vi "Self Starting Simple Frequency Reader.vi"(8 "error in (no error)":errorcluster) -> (0 "error out":errorcluster)   [LabVIEW 2018, in "S3DK.lvlib"]
uses:
  <vilib>/S3DK.lvlib
  <vilib>/Platform/TimedLoop/XDataNode/timing_clust.ctl
  <vilib>/Platform/TimedLoop/XDataNode/nitl_modes.ctl
  <vilib>/Platform/TimedLoop/XDataNode/wakeup.ctl
  <vilib>/platform/TimedLoop/XDataNode/XDataNode.xnode
  <vilib>/Platform/TimedLoop/XDataNode/XDNodeRunTimeDep.lvlib
  .S3DK - Copy/PMU Recorder Light/PMU Recorder Light.lvlib
panel:
  out "Waveform Chart":waveform(sgl)[](graph)
  in  "Quit":bool
  in  "Refresh Rate":i64(ring)=200 items=["50 Hz"=20, "20 Hz"=50, "10 Hz"=100, "5 Hz"=200, "2 Hz"=500, "1 Hz"=1000, "Every 2 sec"=2000, "Every 5 sec"=5000, "Every 10 sec"=10000, "Every minute"=60000]
  # "INPUT"
  # "INTERMEDIATE"
  # "OUTPUT"
  # "USAGE:  Press play. The VI will start the PRL itself and wait for the connection to be established.\n(you will still need to configure the PRL first. If the Simple Frequency Reader works, then this works)"
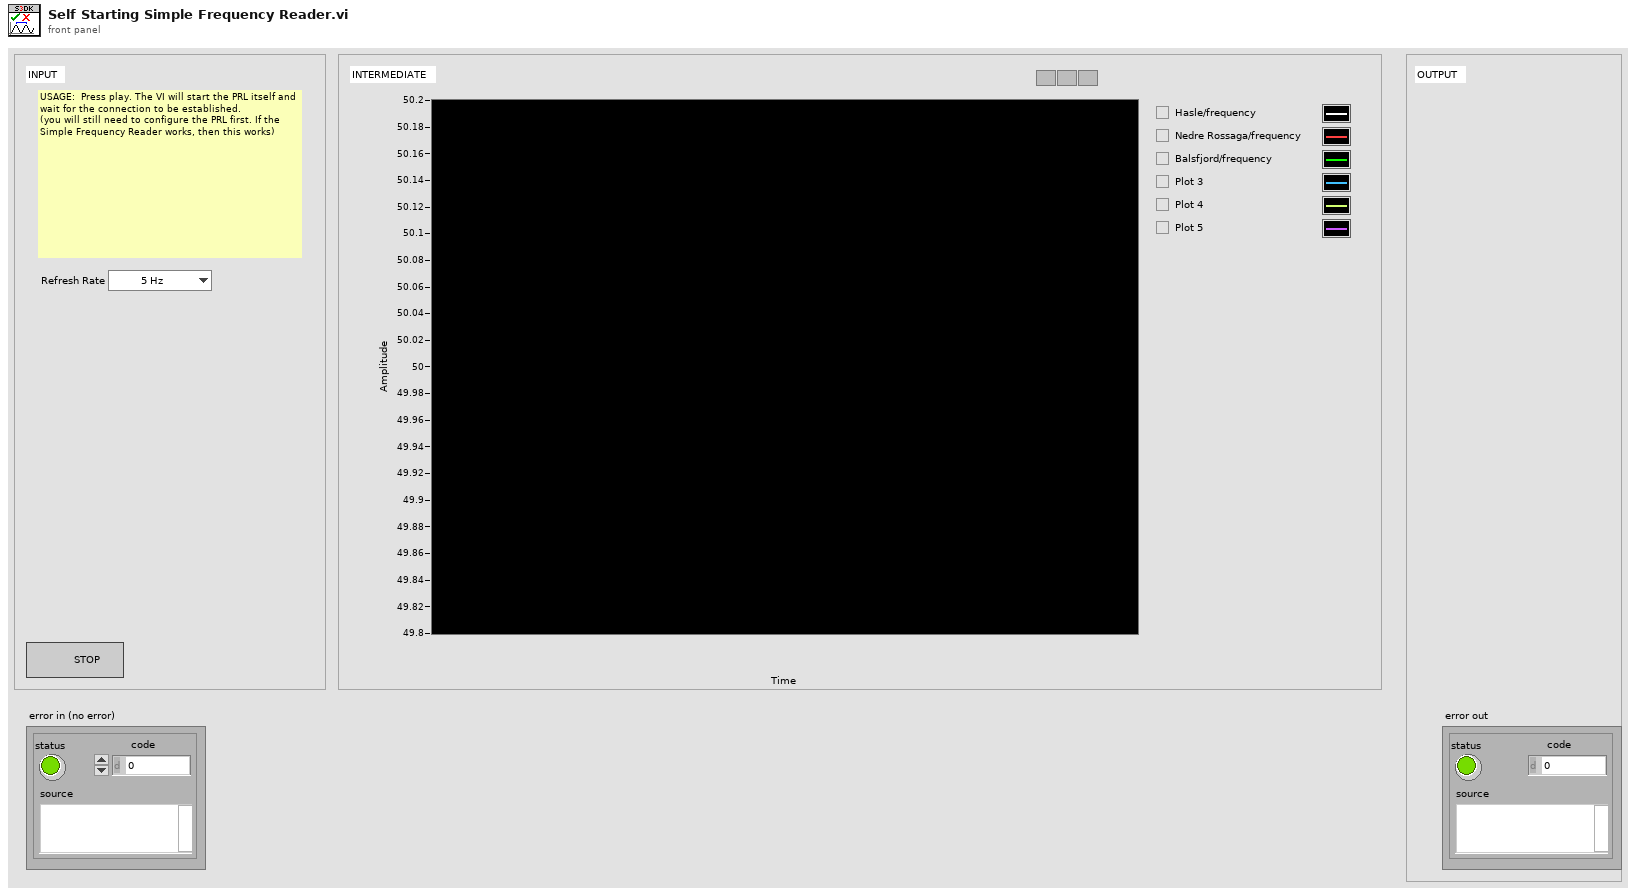
[diagram p1: front panel]
types:
  T1 = enum16{"Run", "Startup", "Get Status", "Pause", "Continue", "Shutdown", "Abort", "Open Panel", "Close Panel"}
  T2 = enum16{"Filter Signals", "Get All Signal Names", "Select Signals on Name", "Select Frequency Only", "Get Selected Signal Names"}
  T3 = typedef "XDNodeRunTimeDep.lvlib/timing_clust.ctl" = cluster{"Expected End [f-1]":u64, "Actual End [f-1]":u64, "Finished Late? [f-1]":bool, "Expected End [i-1]":u64, "Actual End [i-1]":u64, "Finished Late? [i-1]":bool, "Expected Start [i]":u64, "Actual Start [i]":u64, "Expected Start [f]":u64, "Actual Start [f]":u64, "Source Name":string, "Structure Name":string, "Period":i64, "Deadline":i64, "Offset":i64, "Start":i64, "Priority":i32, "Timeout":i32, "Mode":T4, "Wakeup Reason":T5, "Error":errorcluster, "Source Type":string, "Secondary Source Type":string, "Global End Time":u64, "Global Start Time":u64, "Frame Duration":u64, "Iteration Duration":u64, "Assigned CPU":i32, "I/O Scan Engine Mode":u32}
  T4 = typedef "XDNodeRunTimeDep.lvlib/nitl_modes.ctl" = enum32{"No Change", "Process missed periods, maintain original phase", "Discard missed periods, maintain original phase", "Process missed periods, ignore original phase", "Discard missed periods, ignore original phase"}
  T5 = typedef "XDNodeRunTimeDep.lvlib/wakeup.ctl" = enum32{"Normal", "Aborted", "Asynchronous wakeup", "Timing source error", "Timed loop error", "Timeout"}
  T6 = cluster{"Phasor":string[], "Analog":string[], "Digital":string[]}
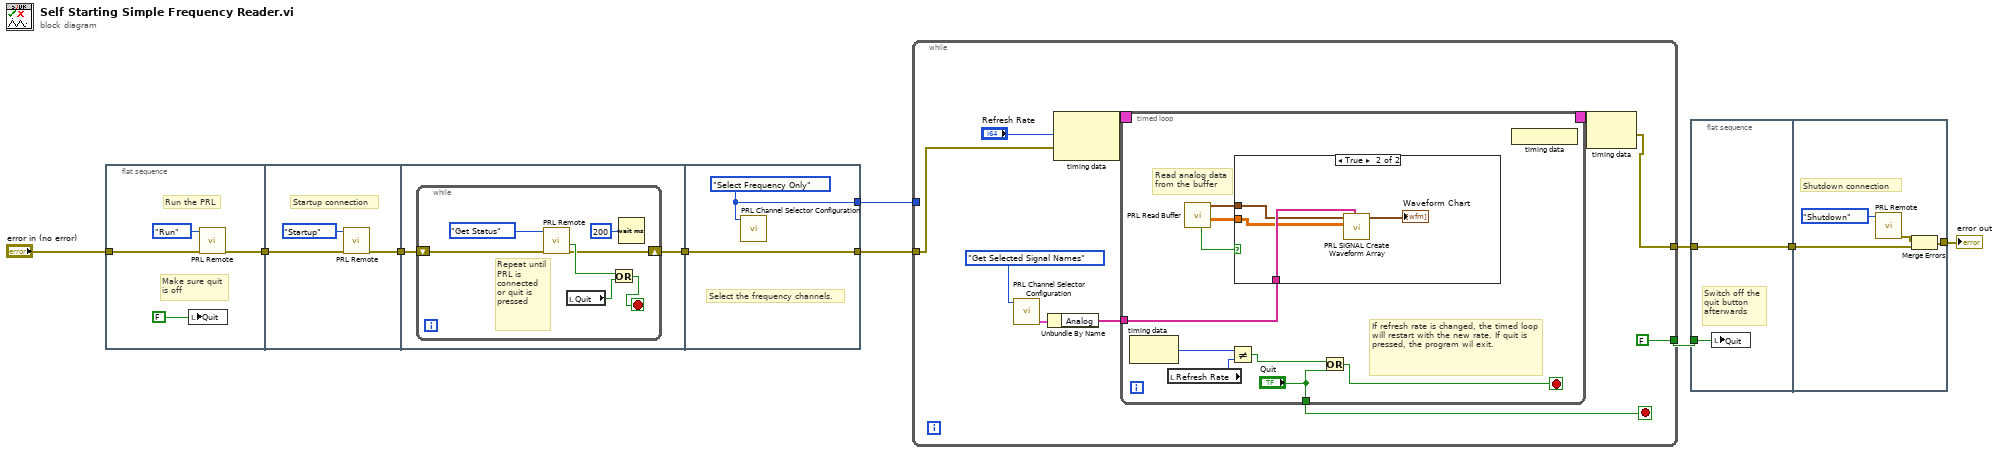
[diagram p0: block diagram]
diagram:
  n1 = flat-sequence {
    tunnel: "error in (no error)" -> [w12]
    tunnel: [w11] -> w7
    tunnel: w7 -> [w16]
    tunnel: [w15] -> w6
    tunnel: w6 -> [w19]
    tunnel: [w18] -> w5
    tunnel: [w28] -> w9
    tunnel: w5 -> [w27]
    tunnel: [w27] -> w4
    frame #0 {
      # "Make sure quit\nis off"
      # "Run the PRL"
      n2 = local write "Quit"(FALSE ("Quit")) -> ()
      n3 = call "PRL Remote.vi"("error in (no error)"=w12, "Action"=T1."Run") -> ("error out"=w11:errorcluster)  [unwired: 4 in, 5 out]
    }
    frame #1 {
      # "Startup connection"
      n4 = call "PRL Remote.vi"("error in (no error)"=w16, "Action"=T1."Startup") -> ("error out"=w15:errorcluster)  [unwired: 4 in, 5 out]
    }
    frame #2 {
      n5 = while {
        shift-right: [w20] -> w18
        shift-left: w19 -> [w21]
        stop <- w24 stop-if-true
        # "Repeat until PRL is connected or quit is pressed"
        n6 = call "PRL Remote.vi"("error in (no error)"=w21, "Action"=T1."Get Status") -> ("error out"=w20:errorcluster, "Connected"=w22:bool)  [unwired: 4 in, 4 out]
        n7 = local read "Quit"() -> (w23:bool)
        n8 = Or(x=w22, y=w23) -> (x .or. y?=w24:bool)
        n9 = Wait (ms)(milliseconds to wait=u32 200) -> ()  [unwired: 1 out]
      }
    }
    frame #3 {
      w28 = T2."Select Frequency Only" ("Action")
      # "Select the frequency channels."
      n10 = call "PRL Channel Selector Configuration.vi"("Action"=w28) -> ()  [unwired: 10 in, 1 out]
    }
  }
  n11 = while {
    tunnel: [FALSE ("Quit")] -> w10
    tunnel: w9 -> [_]
    tunnel: w4 -> [w30]
    tunnel: [w29] -> w2
    stop <- w38 stop-if-true
    n12 = call "PRL Channel Selector Configuration.vi"("Action"=T2."Get Selected Signal Names") -> ("Signal Names Out"=w32:T6)  [unwired: 10 in]
    n13 = Unbundle By Name(w32) -> ("Analog"=w31:string[])
    n14 = node-c288("Refresh Rate", w30) -> (w36:T3)
    n15 = timed-loop {
      timing: w36 -> [_]
      timing-out: [_] -> w35
      tunnel: ["Quit"] -> w38
      tunnel: w31 -> [w39]
      stop <- w45 stop-if-true
      # "Read analog data\nfrom the buffer"
      # "If refresh rate is changed, the timed loop will restart with the new rate. If quit is pressed, the program wil exit."
      n16 = node-c288() -> (w47:i64)  [unwired: 1 in]
      n17 = local read "Refresh Rate"() -> (w46:i64)
      n18 = call "PRL Read Buffer .vi"() -> ("Analog Signals"=w40:sgl[][], "Timestamp"=w41:timestamp[], "Has Data"=w42:bool)  [unwired: 6 in, 3 out]
      n19 = Not Equal?(x=w47, y=w46) -> (x != y?=w44:bool)
      n20 = case shown="True" w42 {
        tunnel: w41 -> [_ w50]
        tunnel: w40 -> [_ w49]
        tunnel: w39 -> [_ w51]
        frame False {
          # "If there is no new data there is no point in sending them to the plot."
        }
        frame True {
          n21 = call "PRL SIGNAL Create Waveform Array.vi"("Signal Names"=w51, "Analog Signals"=w49, "Timestamp"=w50) -> ("Waveform Array"=→"Waveform Chart":waveform(sgl)[])  [unwired: 8 in]
        }
      }
      n22 = Or(x=w44, y="Quit") -> (x .or. y?=w45:bool)
      n23 = node-c288() -> ()  [unwired: 1 out]
    }
    n24 = node-c288(w35) -> (w29:errorcluster)
  }
  n25 = flat-sequence {
    tunnel: w10 -> [w62]
    tunnel: [w61] -> w3
    tunnel: w2 -> [w61]
    tunnel: w3 -> [w64]
    tunnel: [w63] -> w1
    frame #0 {
      # "Switch off the\nquit button\nafterwards"
      n26 = local write "Quit"(w62) -> ()
    }
    frame #1 {
      # "Shutdown connection"
      n27 = call "PRL Remote.vi"("Action"=T1."Shutdown") -> ("error out"=w65:errorcluster)  [unwired: 5 in, 5 out]
      n28 = Merge Errors(w65, w64) -> (w63:errorcluster)
    }
  }
  "error out" <- w1
